vi "parcial tanques.vi"() -> ()   [LabVIEW 2013]
panel:
  out "0%":bool
  out "100%":bool
  out "75%":bool
  out "50%":bool
  out "25%":bool
  out "Tank 2":dbl(slide) scale=0.0..1000.0
  out "100%":bool
  out "90%":bool
  out "80%":bool
  out "70%":bool
  out "60%":bool
  out "50%":bool
  out "40%":bool
  out "30%":bool
  out "20%":bool
  out "10%":bool
  out "Tank 1":dbl(slide) scale=0.0..1000.0
  # "universidad de cundinamarca \ningenieria de  sistemas \nelectiva profesional IV\nandy leandro camargo z"
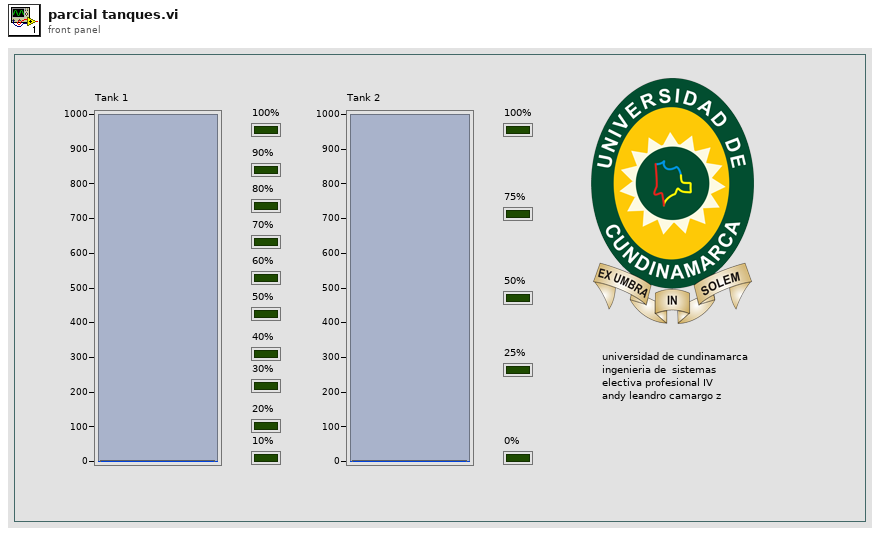
[diagram p1: front panel]
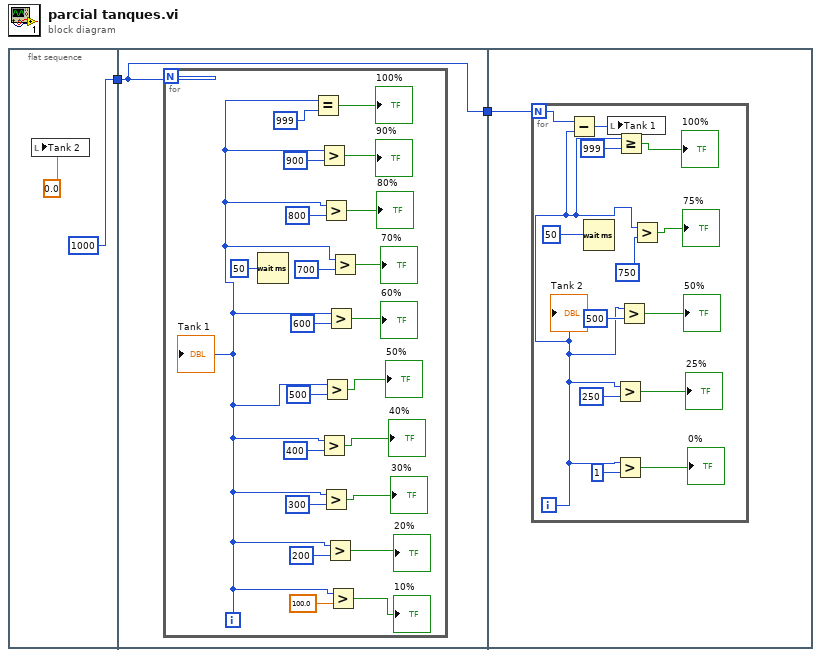
[diagram p0: block diagram]
diagram:
  n1 = flat-sequence {
    tunnel: [1000] -> w2
    tunnel: w2 -> [w5]
    tunnel: [w5] -> w1
    tunnel: w1 -> [w28]
    frame #0 {
      n2 = local write "Tank 2"(0.0 ("Tank 2")) -> ()
    }
    frame #1 {
      n3 = for {
        N: w5 -> [_]
        i -> [w6]
        n4 = Wait (ms)(milliseconds to wait=u32 50) -> ()  [unwired: 1 out]
        n5 = Equal?(x=w6, y=999 ("x")) -> (x = y?=→"100%":bool)
        n6 = Greater?(x=w6, y=900) -> (0:→"90%":bool)
        n7 = Greater?(x=w6, y=400) -> (0:→"40%":bool)
        n8 = Greater?(x=w6, y=800) -> (0:→"80%":bool)
        n9 = Greater?(x=w6, y=300) -> (0:→"30%":bool)
        n10 = Greater?(x=w6, y=500) -> (0:→"50%":bool)
        n11 = Greater?(x=w6, y=200) -> (0:→"20%":bool)
        n12 = Greater?(x=w6, y=600) -> (0:→"60%":bool)
        n13 = Greater?(x=w6, y=100.0) -> (0:→"10%":bool)
        n14 = Greater?(x=w6, y=700) -> (0:→"70%":bool)
        "Tank 1" <- w6
      }
    }
    frame #2 {
      n15 = for {
        N: w28 -> [w31]
        i -> [w30]
        n16 = Subtract(x=w31, y=w30) -> (x-y=w29:i32)
        n17 = Wait (ms)(milliseconds to wait=u32 50 ("millisecond timer value")) -> ()  [unwired: 1 out]
        n18 = local write "Tank 1"(w29) -> ()
        n19 = Greater?(x=w30, y=250) -> (0:→"25%":bool)
        n20 = Greater?(x=w30, y=1) -> (0:→"0%":bool)
        n21 = Greater Or Equal?(x=w30, y=999) -> (x >= y?=→"100%":bool)
        n22 = Greater?(x=w30, y=500) -> (0:→"50%":bool)
        n23 = Greater?(x=w30, y=750) -> (0:→"75%":bool)
        "Tank 2" <- w30
      }
    }
  }
